vi "要求值表格显示.vi"() -> ()   [LabVIEW 2013]
uses:
  <vilib>/Utility/config.llb/Config Data RefNum.ctl
  <vilib>/Utility/config.llb/NI_LVConfig.lvlib
panel:
  out "info":string
  in  "机组":u16(ring) items=["168", "195", "196", "DR96"]
  in  "要求值表格":T1
  in  "stop":bool
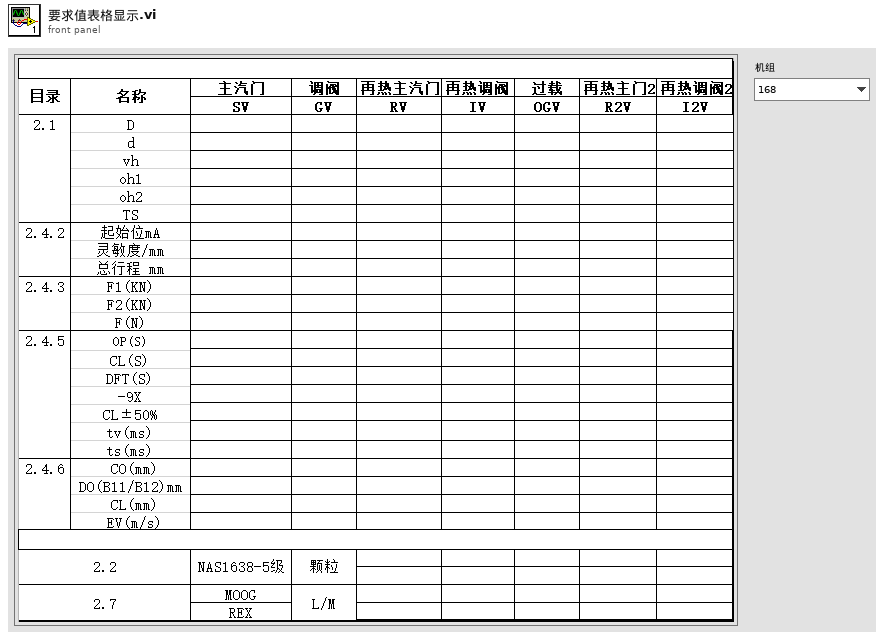
[diagram p1: front panel]
types:
  T1 = cluster{"(GV1)油动机_要求值":string, "字符串 301":string, "2.4.5_OP_SV":string, "2.4.5_OP_GV":string, "2.4.5_OP_RV":string, "2.4.5_OP_IV":string, "2.4.5_OP_OGV":string, "2.4.5_OP_R2V":string, "2.4.5_OP_I2V":string, "2.4.5_CL_SV":string, "2.4.5_CL_GV":string, "2.4.5_CL_RV":string, "2.4.5_CL_IV":string, "2.4.5_CL_OGV":string, "2.4.5_CL_R2V":string, "2.4.5_CL_I2V":string, "2.4.5_DFT_SV":string, "2.4.5_DFT_GV":string, "2.4.5_DFT_RV":string, "2.4.5_DFT_IV":string, "2.4.5_DFT_OGV":string, "2.4.5_DFT_R2V":string, "2.4.5_DFT_I2V":string, "2.4.5_-9X_SV":string, "2.4.5_-9X_GV":string, "2.4.5_-9X_RV":string, "2.4.5_-9X_IV":string, "2.4.5_-9X_OGV":string, "2.4.5_-9X_R2V":string, "2.4.5_-9X_I2V":string, "2.4.5_CL(±50%)_SV":string, "2.4.5_CL(±50%)_GV":string, "2.4.5_CL(±50%)_RV":string, "2.4.5_CL(±50%)_IV":string, "2.4.5_CL(±50%)_OGV":string, "2.4.5_CL(±50%)_R2V":string, "2.4.5_CL(±50%)_I2V":string, "2.4.5_tv_SV":string, "2.4.5_tv_GV":string, "2.4.5_tv_RV":string, "2.4.5_tv_IV":string, "2.4.5_tv_OGV":string, "2.4.5_tv_R2V":string, "2.4.5_tv_I2V":string, "2.4.5_ts_SV":string, "2.4.5_ts_GV":string, "2.4.5_ts_RV":string, "2.4.5_ts_IV":string, "2.4.5_ts_OGV":string, "2.4.5_ts_R2V":string, "2.4.5_ts_I2V":string, "2.4.6_CO_SV":string, "2.4.6_CO_GV":string, "2.4.6_CO_RV":string, "2.4.6_CO_IV":string, "2.4.6_CO_OGV":string, "2.4.6_CO_R2V":string, "2.4.6_CO_I2V":string, "2.4.6_DO_SV":string, "2.4.6_DO_GV":string, "2.4.6_DO_RV":string, "2.4.6_DO_IV":string, "2.4.6_DO_OGV":string, "2.4.6_DO_R2V":string, "2.4.6_DO_I2V":string, "2.4.6_CL_SV":string, "2.4.6_CL_GV":string, "2.4.6_CL_RV":string, "2.4.6_CL_IV":string, "2.4.6_CL_OGV":string, "2.4.6_CL_R2V":string, "2.4.6_CL_I2V":string, "2.4.6_EV_SV":string, "2.4.6_EV_GV":string, "2.4.6_EV_RV":string, "2.4.6_EV_IV":string, "2.4.6_EV_OGV":string, "2.4.6_EV_R2V":string, "2.4.6_EV_I2V":string, "2.2_颗粒_1_SV":string, "2.2_颗粒_1_GV":string, "2.2_颗粒_1_RV":string, "2.2_颗粒_1_IV":string, "2.2_颗粒_1_OGV":string, "2.2_颗粒_2_SV":string, "2.2_颗粒_2_GV":string, "2.2_颗粒_2_RV":string, "2.2_颗粒_2_IV":string, "2.2_颗粒_2_OGV":string, "2.7_L/M_1_SV":string, "2.7_L/M_1_GV":string, "2.7_L/M_1_RV":string, "2.7_L/M_1_IV":string, "2.7_L/M_1_OGV":string, "2.7_L/M_2_SV":string, "2.7_L/M_2_GV":string, "2.7_L/M_2_RV":string, "2.7_L/M_2_IV":string, "2.7_L/M_2_OGV":string, "2.1_D_SV":string, "2.1_D_GV":string, "2.1_D_RV":string, "2.1_D_IV":string, "2.1_D_OGV":string, "2.1_D_R2V":string, "2.1_D_I2V":string, "2.1_d0_SV":string, "2.1_d0_GV":string, "2.1_d0_RV":string, "2.1_d0_IV":string, "2.1_d0_OGV":string, "2.1_d0_R2V":string, "2.1_d0_I2V":string, "2.1_vh_SV":string, "2.1_vh_GV":string, "2.1_vh_RV":string, "2.1_vh_IV":string, "2.1_vh_OGV":string, "2.1_vh_R2V":string, "2.1_vh_I2V":string, "2.1_oh1_SV":string, "2.1_oh1_GV":string, "2.1_oh1_RV":string, "2.1_oh1_IV":string, "2.1_oh1_OGV":string, "2.1_oh1_R2V":string, "2.1_oh1_I2V":string, "2.1_oh2_SV":string, "2.1_oh2_GV":string, "2.1_oh2_RV":string, "2.1_oh2_IV":string, "2.1_oh2_OGV":string, "2.1_oh2_R2V":string, "2.1_oh2_I2V":string, "2.1_TS_SV":string, "2.1_TS_GV":string, "2.1_TS_RV":string, "2.1_TS_IV":string, "2.1_TS_OGV":string, "2.1_TS_R2V":string, "2.1_TS_I2V":string, "2.4.2_起始位_SV":string, "2.4.2_灵敏度_SV":string, "2.4.2_总行程_SV":string, "2.4.2_起始位_GV":string, "2.4.2_起始位_RV":string, "2.4.2_起始位_IV":string, "2.4.2_起始位_OGV":string, "2.4.2_起始位_R2V":string, "2.4.2_起始位_I2V":string, "2.4.2_灵敏度_GV":string, "2.4.2_灵敏度_RV":string, "2.4.2_灵敏度_IV":string, "2.4.2_灵敏度_OGV":string, "2.4.2_灵敏度_R2V":string, "2.4.2_灵敏度_I2V":string, "2.4.2_总行程_GV":string, "2.4.2_总行程_RV":string, "2.4.2_总行程_IV":string, "2.4.2_总行程_OGV":string, "2.4.2_总行程_R2V":string, "2.4.2_总行程_I2V":string, "2.4.3_F1_GV":string, "2.4.3_F1_RV":string, "2.4.3_F1_IV":string, "2.4.3_F1_OGV":string, "2.4.3_F1_R2V":string, "2.4.3_F1_I2V":string, "2.4.3_F2_GV":string, "2.4.3_F2_RV":string, "2.4.3_F2_IV":string, "2.4.3_F2_OGV":string, "2.4.3_F2_R2V":string, "2.4.3_F2_I2V":string, "2.4.3_F_GV":string, "2.4.3_F_RV":string, "2.4.3_F_IV":string, "2.4.3_F_OGV":string, "2.4.3_F_R2V":string, "2.4.3_F_I2V":string, "2.4.3_F1_SV":string, "2.4.3_F2_SV":string, "2.4.3_F_SV":string}
  T2 = typedef "NI_LVConfig.lvlib/Config Data RefNum.ctl" = refnum<k1>
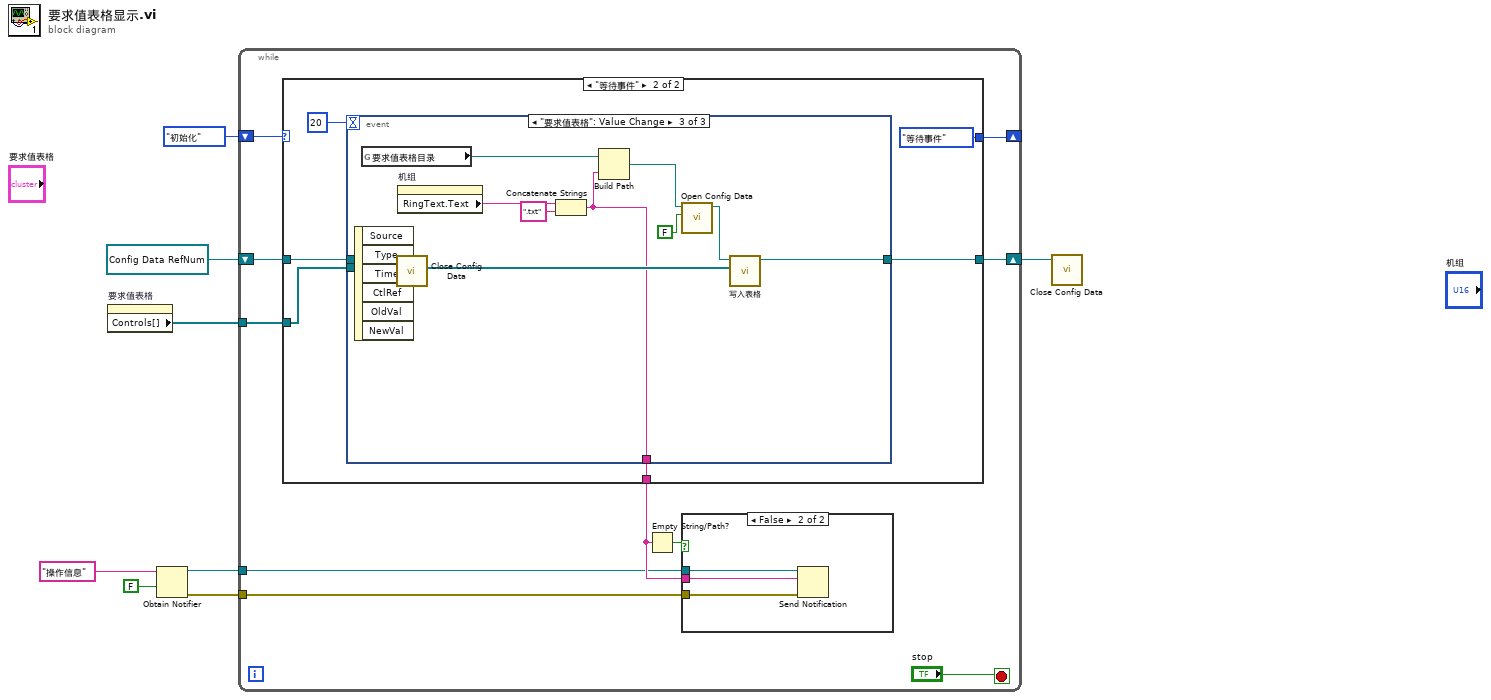
[diagram p0: block diagram]
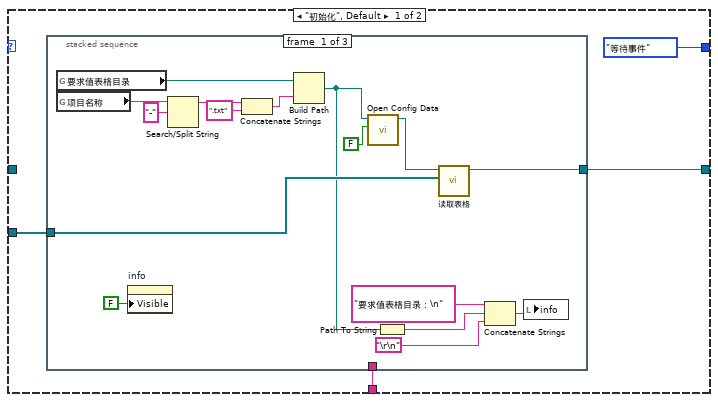
[diagram p3: hidden frame]
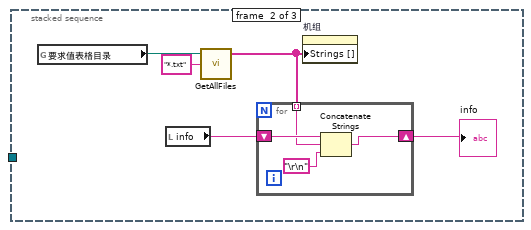
[diagram p4: hidden frame]
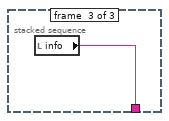
[diagram p5: hidden frame]
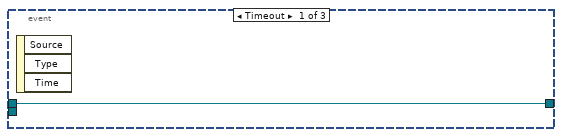
[diagram p6: hidden frame]
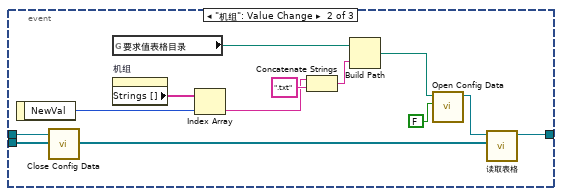
[diagram p7: hidden frame]
diagram:
  w4 = "操作信息"
  w7 = T2 refnum items=["config data"] ("引用句柄输入")
  n1 = property on="要求值表格" class="Clust (strict)"() -> ("Controls[]"=w5:refnum<vi>[])  [unwired: 2 in, 2 out]
  n2 = Obtain Notifier(name (unnamed)=w4, notification data type=w4, create if not found? (T)=FALSE) -> (notifier out=w2:refnum<notifier>, error out=w1:errorcluster)  [unwired: 1 in, 1 out]
  n3 = while {
    shift-right: [w16] -> _
    shift-left: enum16{"初始化", "等待事件"}."初始化" -> [w17]
    shift-right: [w15] -> w8
    shift-left: w7 -> [w13]
    tunnel: w5 -> [w14]
    tunnel: w2 -> [w10]
    tunnel: w1 -> [w9]
    stop <- "stop" stop-if-true
    n4 = case shown="\"等待事件\"" w17 {
      tunnel: [enum16{"初始化", "等待事件"}."等待事件" enum16{"初始化", "等待事件"}."等待事件"] -> w16
      tunnel: [w24 w53] -> w15
      tunnel: w14 -> [w23 w55]
      tunnel: w13 -> [_ w54]
      tunnel: [w22 w52] -> w11
      frame "初始化", Default {
        n5 = stacked-sequence {
          tunnel: [w39 _ _] -> w24
          tunnel: w23 -> [w38 _ _]
          tunnel: [_ _ w51] -> w22
          frame #0 {
            n6 = global read "要求值表格目录.vi" "要求值表格目录"() -> (w33:path)
            n7 = global read "项目名称.vi" "项目名称"() -> (w37:string)
            n8 = property on="info" class="Str"("Visible"=FALSE) -> ()  [unwired: 2 in, 2 out]
            n9 = Search/Split String(string=w37, search string/char (-)="-") -> (substring before match=w35:string)  [unwired: 1 in, 2 out]
            n10 = Concatenate Strings(w35, ".txt" ("string")) -> (w32:string)
            n11 = Build Path(base path=w33, name or relative path=w32) -> (appended path=w30:path)
            n12 = call <vilib>:"Open Config Data.vi"("create file if necessary (T)"=FALSE, "configuration file path"=w30) -> ("refnum"=w40:T2)  [unwired: 7 in, 2 out]
            n13 = Path To String(path=w30) -> (string=w29:string)
            n14 = call "读取表格.vi"("Controls[]"=w38, "引用句柄输入"=w40) -> ("引用句柄输出"=w39:T2)  [unwired: 8 in, 1 out]
            n15 = Concatenate Strings("要求值表格目录：\n", w29, "\r\n") -> (w28:string)
            n16 = local write "info"(w28) -> ()
          }
          frame #1 {
            n17 = global read "要求值表格目录.vi" "要求值表格目录"() -> (w46:path)
            n18 = local read "info"() -> (w43:string)
            n19 = call "GetAllFiles.vi"("Pattern"="*.txt", "FolderPath"=w46) -> ("Files"=w44:string[])  [unwired: 2 in, 1 out]
            n20 = for {
              shift-right: [w47] -> w42
              shift-left: w43 -> [w49]
              tunnel: w44 -> [w48] mode=indexing
              n21 = Concatenate Strings(w49, w48, "\r\n") -> (w47:string)
            }
            "info" <- w42
            n22 = property on="机组" class="Ring (strict)"("Strings []"=w44) -> ()  [unwired: 2 in, 2 out]
          }
          frame #2 {
            n23 = local read "info"() -> (w51:string)
          }
        }
      }
      frame "等待事件" {
        n24 = event shown="[2] \"要求值表格\": Value Change" {
          selector: _ -> [_ _ _]
          dyn-events: _ -> [_ _ _]
          timeout: 20 -> [_ _ _]
          tunnel: w55 -> [_ w61 w80]
          tunnel: w54 -> [w58 w59 w74]
          tunnel: [w58 w60 w71] -> w53
          tunnel: [_ _ w72] -> w52
          event Timeout {
            n25 = event-data() -> ()  [unwired: 1 in, 3 out]
          }
          event "机组": Value Change {
            n26 = event-data() -> ("NewVal"=w69:u16)  [unwired: 1 in]
            n27 = call <vilib>:"Close Config Data.vi"("refnum"=w59) -> ()  [unwired: 9 in, 2 out]
            n28 = global read "要求值表格目录.vi" "要求值表格目录"() -> (w63:path)
            n29 = property on="机组" class="Ring (strict)"() -> ("Strings []"=w70:string[])  [unwired: 2 in, 2 out]
            n30 = Index Array(array=w70, index=w69) -> (element=w62:string)
            n31 = Concatenate Strings(w62, ".txt" ("string")) -> (w67:string)
            n32 = Build Path(base path=w63, name or relative path=w67) -> (appended path=w68:path)
            n33 = call <vilib>:"Open Config Data.vi"("create file if necessary (T)"=FALSE, "configuration file path"=w68) -> ("refnum"=w65:T2)  [unwired: 7 in, 2 out]
            n34 = call "读取表格.vi"("Controls[]"=w61, "引用句柄输入"=w65) -> ("引用句柄输出"=w60:T2)  [unwired: 8 in, 1 out]
          }
          event "要求值表格": Value Change {
            n35 = event-data() -> ()  [unwired: 1 in, 6 out]
            n36 = global read "要求值表格目录.vi" "要求值表格目录"() -> (w76:path)
            n37 = call <vilib>:"Close Config Data.vi"("refnum"=w74) -> ()  [unwired: 9 in, 2 out]
            n38 = property on="机组" class="Ring (strict)"() -> ("RingText.Text"=w73:string)  [unwired: 2 in, 2 out]
            n39 = Concatenate Strings(w73, ".txt" ("string")) -> (w72:string)
            n40 = Build Path(base path=w76, name or relative path=w72) -> (appended path=w79:path)
            n41 = call <vilib>:"Open Config Data.vi"("create file if necessary (T)"=FALSE, "configuration file path"=w79) -> ("refnum"=w75:T2)  [unwired: 7 in, 2 out]
            n42 = call "写入表格.vi"("Controls[]"=w80, "引用句柄输入"=w75) -> ("引用句柄输出"=w71:T2)  [unwired: 8 in, 1 out]
          }
        }
      }
    }
    n43 = Empty String/Path?(string/path=w11) -> (empty?=w12:bool)
    n44 = case shown="False" w12 {
      tunnel: w10 -> [_ w21]
      tunnel: w9 -> [_ w20]
      tunnel: w11 -> [_ w19]
      frame True {
      }
      frame False {
        n45 = Send Notification(notification=w19, notifier=w21, error in (no error)=w20) -> ()  [unwired: 2 out]
      }
    }
  }
  n46 = call <vilib>:"Close Config Data.vi"("refnum"=w8) -> ()  [unwired: 9 in, 2 out]
